vi "Configure Output.vi"(8 "error in (no error)":errorcluster, 10 "Voltage Level (0.0 V)":dbl format="%.3g", 11 "VISA resource name":refnum<visa-resource-name>) -> (0 "error out":errorcluster, 3 "VISA resource name out":refnum<visa-resource-name>)   [LabVIEW 2021, in "BK Precision 9200 Series.lvlib"]
doc: "Configures output voltage level output of the power supply."
uses:
  <instrlib>/BK Precision 9200 Series/BK Precision 9200 Series.lvlib
panel:
  # "V"
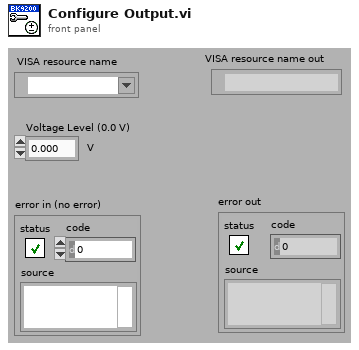
[diagram p1: front panel]
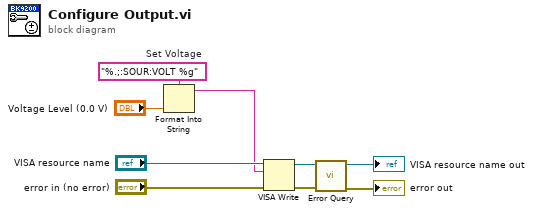
[diagram p0: block diagram]
diagram:
  w7 = "%.;:SOUR:VOLT %g"  # Set Voltage
  n1 = Format Into String(format string=w7, "Voltage Level (0.0 V)") -> (resulting string=w1:string)  [unwired: 2 in, 1 out]
  n2 = VISA Write(VISA resource name="VISA resource name", write buffer=w1, error in (no error)="error in (no error)") -> (VISA resource name out=w5:refnum<visa-resource-name>, error out=w4:errorcluster)  [unwired: 1 out]
  n3 = call <instrlib>:"Error Query.vi"("error in (no error)"=w4, "VISA resource name"=w5) -> ("error out"=→"error out":errorcluster, "VISA resource name out"=→"VISA resource name out":refnum<visa-resource-name>)  [unwired: 6 in, 2 out]
